vi "Pass If Error.vi"(7 "Description":string, 8 "error in (no error)":errorcluster, 10 "Assert error":errorcluster, 11 "LUnit Test Case In":refnum<class "LUnit Test Case.lvclass">) -> (0 "error out":errorcluster, 3 "LUnit Test Case Out":refnum<class "LUnit Test Case.lvclass">)   [LabVIEW 2020, in "LUnit Test Case.lvclass"]
doc: "Generates a pass result for the calling test method if the inputs contains an error with status \"True\". A description may be provided to the result."
uses:
  LUnit Test Case.lvclass
  Result Types/Assertion Result/Public/TypeDefs/Assertion Type.ctl
  LUnit Test Case.lvclass/LUnit Test Case.ctl
  Private/SubVIs/Add test result.vi
  Result Types/Case Result/Public/Record Assertion Result.vi
  Result Types/Method Result/Public/Aggregate Assertion Results.vi
  Result Types/Method Result/Private/Merge Status.vi
  Result Types/Method Result/Private/Concatenate result strings.vi
  Result Types/Assertion Result/Assertion Result.lvlib
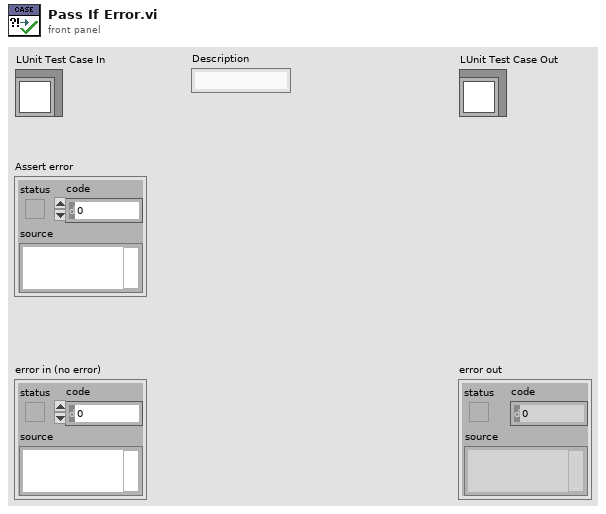
[diagram p1: front panel]
types:
  T1 = typedef "Assertion Result.lvlib/Assertion Type.ctl" = enum16{"None", "Pass", "Fail", "Skip", "Pass if Equal", "Fail if Equal", "Pass if Error", "Fail if Error", "Pass if", "Fail if"}
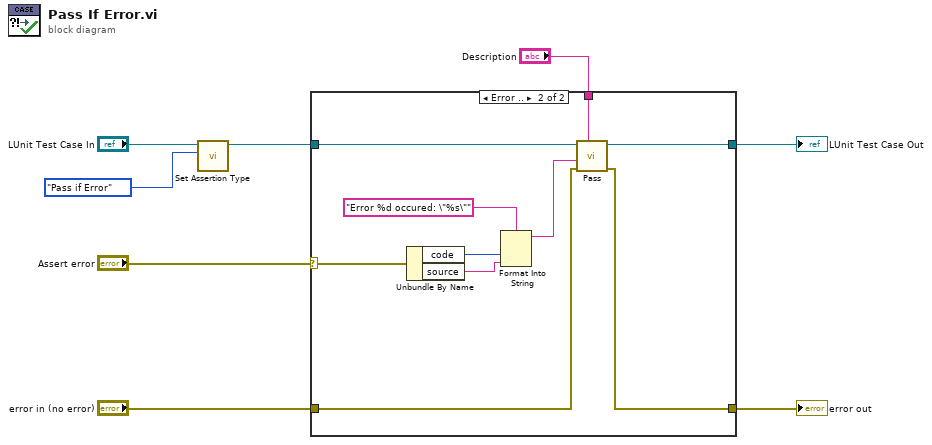
[diagram p0: block diagram]
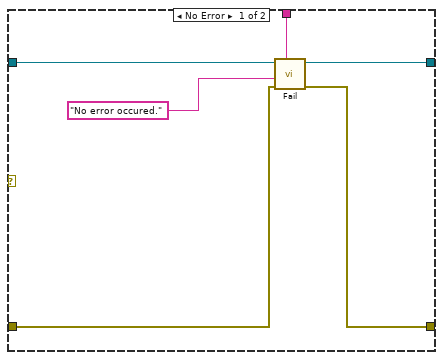
[diagram p2: hidden frame]
diagram:
  n1 = call "Set Assertion Type.vi"("Assertion Type"=Assertion_Type."Pass if Error", "LUnit Test Case In"="LUnit Test Case In") -> ("LUnit Test Case Out"=w3:refnum<class "LUnit Test Case.lvclass">)  [unwired: 9 in]
  n2 = case shown="Error .." "Assert error" {
    selector: "Assert error" -> [_ w21]
    tunnel: w3 -> [w14 w24]
    tunnel: [w13 w23] -> w6
    tunnel: [w12 w22] -> w5
    tunnel: "Description" -> [w11 w19]
    tunnel: "error in (no error)" -> [w9 w15]
    frame No Error {
      n3 = call "Fail.vi"("Description"=w11, "error in (no error)"=w9, "Message"="No error occured.", "LUnit Test Case In"=w14) -> ("error out"=w12:errorcluster, "LUnit Test Case Out"=w13:refnum<class "LUnit Test Case.lvclass">)  [unwired: 6 in]
    }
    frame Error {
      n4 = Unbundle By Name(w21) -> ("code"=w17:i32, "source"=w16:string)
      n5 = Format Into String(format string="Error %d occured: \"%s\"", w17, w16) -> (resulting string=w20:string)  [unwired: 2 in, 1 out]
      n6 = call "Pass.vi"("Description"=w19, "error in (no error)"=w15, "Message"=w20, "LUnit Test Case In"=w24) -> ("error out"=w22:errorcluster, "LUnit Test Case Out"=w23:refnum<class "LUnit Test Case.lvclass">)  [unwired: 6 in]
    }
  }
  "error out" <- w5
  "LUnit Test Case Out" <- w6
